vi "AnyBuilderBeginNestedMessage.vi"(8 "error in":errorcluster, 10 "protobufId":i32, 11 "gRPCid in":T1) -> (0 "error out":errorcluster, 2 "Nested ID":T1, 3 "gRPCid out":T1)   [LabVIEW 2019, in "grpc-lvsupport.lvlib"]
uses:
  grpc-lvsupport.lvlib
  grpcId.ctl
  <vilib>/Utility/error.llb/Error Cluster From Error Code.vi
  <resource>/labview_grpc_server.dll
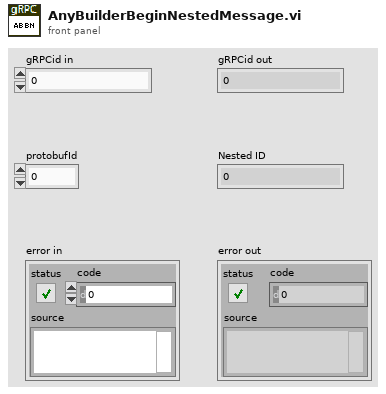
[diagram p1: front panel]
types:
  T1 = typedef "grpc-lvsupport.lvlib/grpcId.ctl" = u64
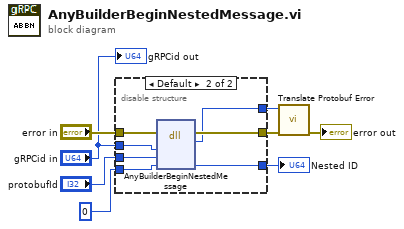
[diagram p0: block diagram]
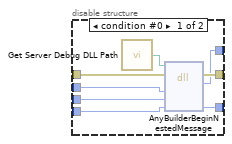
[diagram p2: hidden frame]
diagram:
  n1 = disable-structure shown="Default" {
    disable-tunnel: "error in" -> [w16 w23]
    disable-tunnel: [w15 w22] -> w7
    disable-tunnel: "protobufId" -> [w14 w21]
    disable-tunnel: "gRPCid in" -> [w13 w20]
    disable-tunnel: [w11 w19] -> w5
    disable-tunnel: u64 0 ("nestedId") -> [w10 w18]
    disable-tunnel: [w9 w17] -> w2
    frame condition #0 {
      n2 = call "Get Server Debug DLL Path.vi"() -> ("DLL Path"=w12:path)
      n3 = dll-call lib="?" fn="AnyBuilderBeginNestedMessage"(path in=w12, error in=w16, "builderId"=w13, "protobufId"=w14, "nestedId"=w10) -> (error out=w15:errorcluster, "return type"=w9:i32, "nestedId"=w11:u64)  [unwired: 3 in, 1 out]
    }
    frame condition #1 (active) {
      n4 = dll-call lib="C:/Program Files (x86)/National Instruments/LabVIEW 2024/resource/labview_grpc_server.*" fn="AnyBuilderBeginNestedMessage"(error in=w23, "builderId"=w20, "protobufId"=w21, "nestedId"=w18) -> (error out=w22:errorcluster, "return type"=w17:i32, "nestedId"=w19:u64)  [unwired: 4 in, 1 out]
    }
  }
  "Nested ID" <- w5
  n5 = call "Translate Protobuf Error.vi"("error in"=w7, "Error Code"=w2) -> ("error out"=→"error out":errorcluster)  [unwired: 9 in]
  "gRPCid out" <- "gRPCid in"
